vi "VI Server_CloseRefs.vi"(8 "error in":errorcluster, 11 "VI Server.RefsCluster":T1) -> (0 "error out":errorcluster)   [LabVIEW 2020]
uses:
  VI Server_TypeDefs/VI Server_RefsCluster.ctl
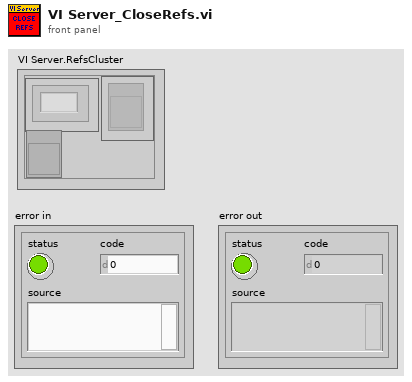
[diagram p1: front panel]
types:
  T1 = typedef "VI Server_RefsCluster.ctl" = cluster{"Labels":string[], "Refs":refnum<vi>[], "VI Ref":refnum<vi>}
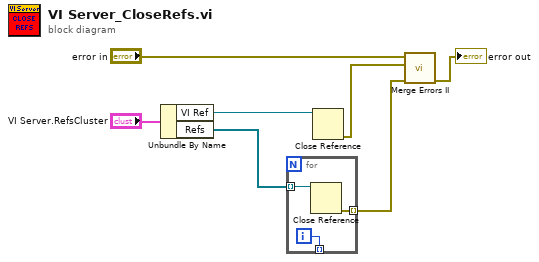
[diagram p0: block diagram]
diagram:
  n1 = Unbundle By Name("VI Server.RefsCluster") -> ("VI Ref"=w6:refnum<vi>, "Refs"=w2:refnum<vi>[])
  n2 = for {
    tunnel: w2 -> [w9] mode=indexing
    tunnel: [w10] -> w1 mode=indexing
    tunnel: [w8] -> _ mode=indexing
    i -> [w8]
    n3 = Close Reference(reference=w9) -> (error out=w10:errorcluster)  [unwired: 1 in]
  }
  n4 = Close Reference(reference=w6) -> (error out=w3:errorcluster)  [unwired: 1 in]
  n5 = call "Merge Errors II.vi"("error array in"=w1, "error in 2 (no error)"=w3, "error in 1 (no error)"="error in") -> ("error out"=→"error out":errorcluster)  [unwired: 3 in, 1 out]
